vi "Regular Waves (DAQmx).vi"(0 "Run":bool, 1 "Wave Period":dbl(slide)=1.0 min=0.5 max=5.0 step=0.01 scale=0.5..5.0 scale format="%.1f", 2 "Wave Height":dbl(slide)=0.1 min=0.0 step=0.001 scale=0.0..0.2869843515506789 scale format="%.3f") -> ()   [LabVIEW 2012]
uses:
  <vilib>/Analysis/1siggen.llb/Ramp Pattern by Samples.vi
  <vilib>/Analysis/NI_AALBase.lvlib
panel:
  out "Waveform Graph":dbl[](graph)
  out "Waveform Chart":dbl[][](graph)
  in  "Measure Waves":bool
  in  "Settings":bool
  in  "Power":bool
  out "Buffer Size":i32=4000
  # "Regular Wave Generator"
  # "s"
  # "m"
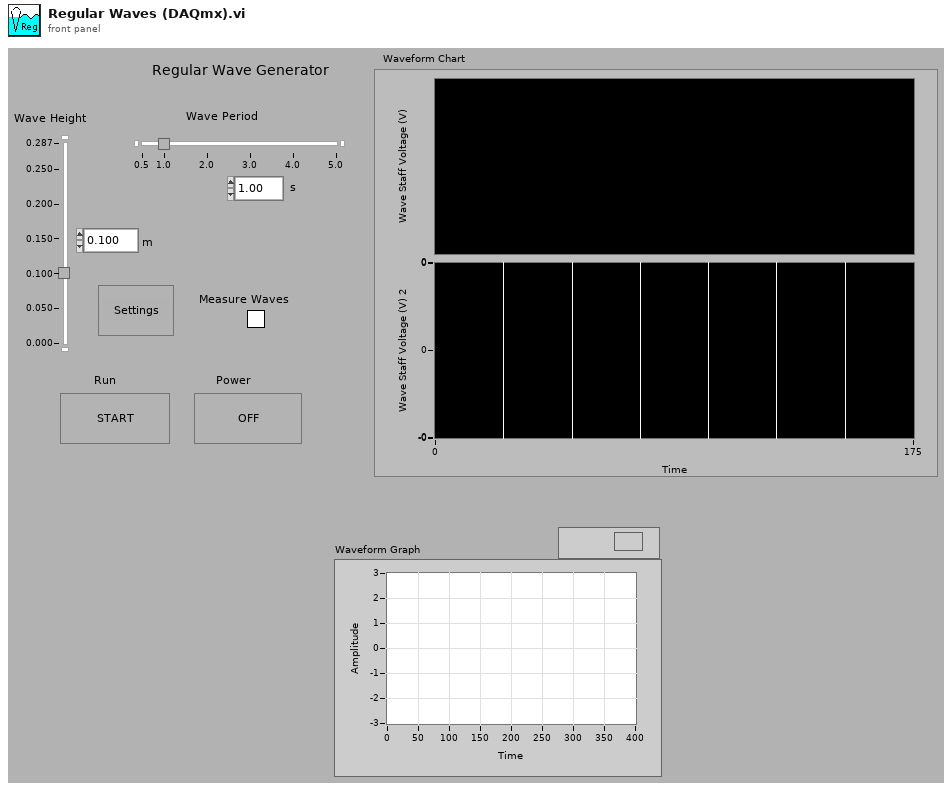
[diagram p1: front panel]
types:
  T1 = cluster{"Output Device":i16, "Output Channel":string, "Sampling Rate (Hz)":dbl, "Input Device":i16, "Input Channel":string, "Input Offset (V)":dbl, "Input Calibration (m/V)":dbl, "Stroke Calibration (V/m)":dbl, "Paddle Height (m)":dbl, "Water Depth (m)":dbl, "Min Period":dbl, "Max Period":dbl, "Max 1/2 Piston Stroke":dbl, "Max H/L":dbl, "Max H/d":dbl}
  T2 = cluster{"Period":dbl, "Wave Height":dbl, "Phase Angle (rad)":dbl}
  T3 = cluster{"Sampling Rate":i32, "Water Depth":dbl, "Paddle Height":dbl}
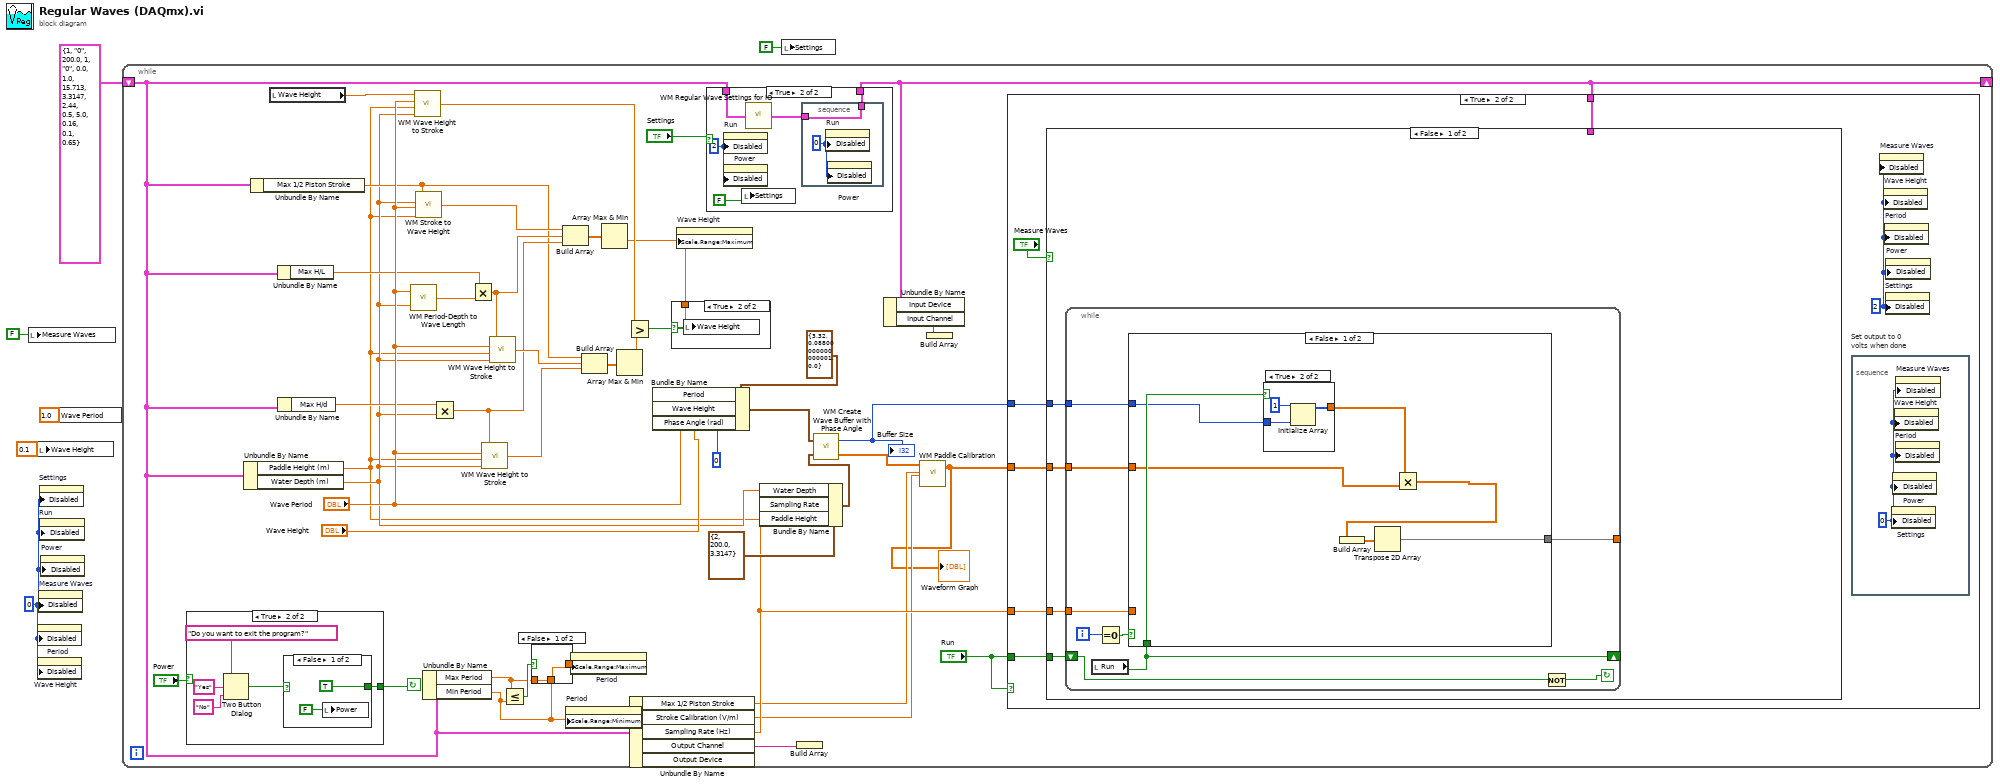
[diagram p0: block diagram]
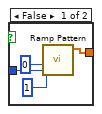
[diagram p3: hidden frame]
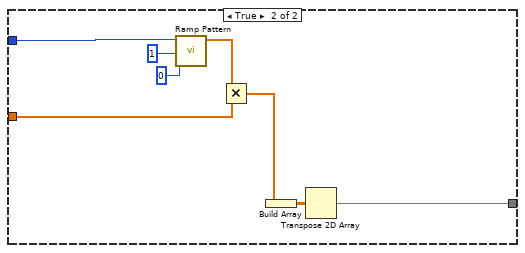
[diagram p4: hidden frame]
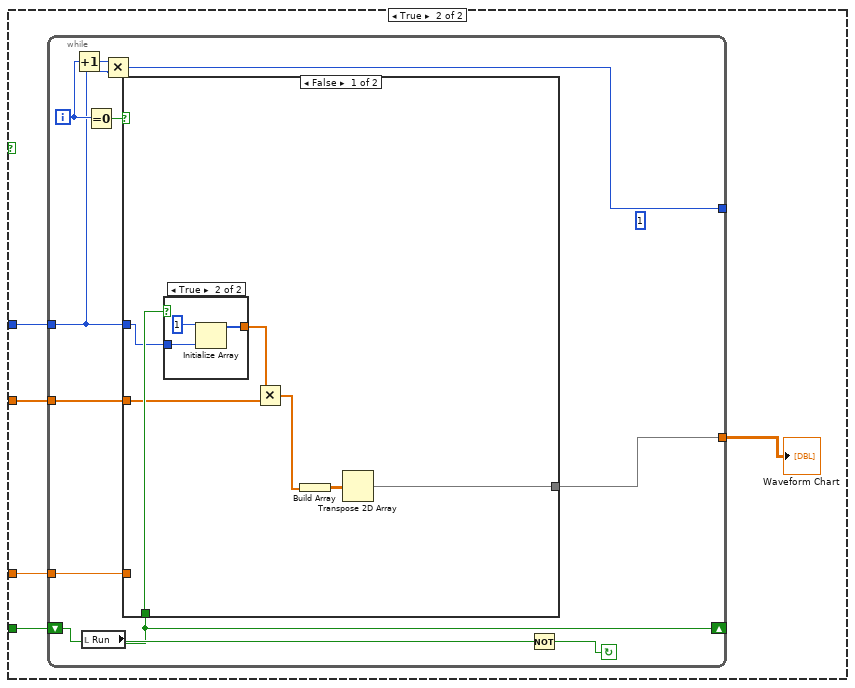
[diagram p5: hidden frame]
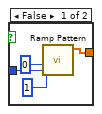
[diagram p6: hidden frame]
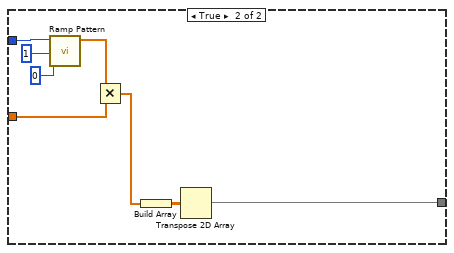
[diagram p7: hidden frame]
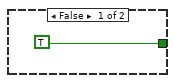
[diagram p9: hidden frame]
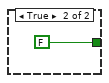
[diagram p10: hidden frame]
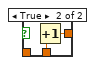
[diagram p11: hidden frame]
diagram:
  w2 = u8 0 ("Write Attribute")
  n1 = local write "Measure Waves"(FALSE ("Measure Waves")) -> ()
  n2 = local write "Wave Height"(0.1 ("Wave Height")) -> ()
  n3 = property on="Period" class="Slide (strict)"("Disabled"=w2) -> ()  [unwired: 2 in, 2 out]
  n4 = property on="Wave Height" class="Slide (strict)"("Disabled"=w2) -> ()  [unwired: 2 in, 2 out]
  n5 = property on="Measure Waves" class="Bool (strict)"("Disabled"=w2) -> ()  [unwired: 2 in, 2 out]
  n6 = property on="Settings" class="Bool (strict)"("Disabled"=w2) -> ()  [unwired: 2 in, 2 out]
  n7 = property on="Run" class="Bool (strict)"("Disabled"=w2) -> ()  [unwired: 2 in, 2 out]
  n8 = property on="Power" class="Bool (strict)"("Disabled"=w2) -> ()  [unwired: 2 in, 2 out]
  n9 = local write "Wave Period"(1.0 ("Period")) -> ()
  n10 = while {
    shift-left: T1 {"Output Device"=1, "Output Channel"="0", "Sampling Rate (Hz)"=200.0, "Input Device"=1, "Input Channel"="0", "Input Offset (V)"=0.0, "Input Calibration (m/V)"=1.0, "Stroke Calibration (V/m)"=15.713, "Paddle Height (m)"=3.3147, "Water Depth (m)"=2.44, "Min Period"=0.5, "Max Period"=5.0, "Max 1/2 Piston Stroke"=0.16, "Max H/L"=0.1, "Max H/d"=0.65} ("Settings") -> [w15]
    shift-right: [w9] -> _
    stop <- w35 continue-if-true
    n11 = case shown="True" "Power" {
      tunnel: [TRUE w140] -> w35
      frame False {
      }
      frame True {
        n12 = Two Button Dialog(message="Do you want to exit the program?", 1:"No" ("F button name (\"Cancel\")"), 2:"Yes" ("T button name (\"OK\")")) -> (T button?=w141:bool)
        n13 = case shown="False" w141 {
          tunnel: [TRUE FALSE] -> w140
          frame False {
            n14 = local write "Power"(FALSE ("Power")) -> ()
          }
          frame True {
          }
        }
      }
    }
    n15 = Unbundle By Name(w15) -> ("Paddle Height (m)"=w18:dbl, "Water Depth (m)"=w19:dbl)
    n16 = Unbundle By Name(w15) -> ("Max 1/2 Piston Stroke"=w22:dbl)
    n17 = local read "Wave Height"() -> (w38:dbl)
    n18 = Unbundle By Name(w15) -> ("Max H/L"=w21:dbl)
    n19 = Unbundle By Name(w15) -> ("Max H/d"=w20:dbl)
    n20 = call "WM Period-Depth to Wave Length.vi"("Water Depth"=w19, "Period"="Wave Period") -> ("WaveLength"=w28:dbl)
    n21 = call "WM Wave Height to Stroke.vi"("Water Depth (m)"=w19, "Flap Height (m)"=w18, "Wave Period (s)"="Wave Period", "Wave Height (m)"=w38) -> ("Flap Amplitude (from x=0) (m)"=w47:dbl)
    n22 = call "WM Stroke to Wave Height.vi"("Paddle Height (m)"=w18, "Wave Period (s)"="Wave Period", "Water Depth (m)"=w19, "Flap Amplitude from x=0 (m)"=w22) -> ("Wave Height (m)"=w42:dbl)
    n23 = Unbundle By Name(w15) -> ("Max Period"=w14:dbl, "Min Period"=w13:dbl)
    n24 = Multiply(x=w20, y=w19) -> (x*y=w27:dbl)
    n25 = Multiply(x=w21, y=w28) -> (x*y=w43:dbl)
    n26 = call "WM Wave Height to Stroke.vi"("Water Depth (m)"=w19, "Flap Height (m)"=w18, "Wave Period (s)"="Wave Period", "Wave Height (m)"=w27) -> ("Flap Amplitude (from x=0) (m)"=w41:dbl)
    n27 = call "WM Wave Height to Stroke.vi"("Water Depth (m)"=w19, "Flap Height (m)"=w18, "Wave Period (s)"="Wave Period", "Wave Height (m)"=w43) -> ("Flap Amplitude (from x=0) (m)"=w40:dbl)
    n28 = Less Or Equal?(x=w14, y=w13) -> (x <= y?=w48:bool)
    n29 = case shown="False" w48 {
      tunnel: w13 -> [_ w150]
      tunnel: [w148 w149] -> w37
      tunnel: w14 -> [w148 _]
      frame False {
      }
      frame True {
        n30 = Increment(x=w150) -> (x+1=w149:dbl)
      }
    }
    n31 = Build Array(w42, w43, w27) -> (w46:dbl[])
    n32 = property on="Period" class="Slide (strict)"("Scale.Range:Minimum"=w13) -> ()  [unwired: 2 in, 2 out]
    n33 = property on="Period" class="Slide (strict)"("Scale.Range:Maximum"=w37) -> ()  [unwired: 2 in, 2 out]
    n34 = Build Array(w22, w40, w41) -> (w45:dbl[])
    n35 = Array Max & Min(array=w46) -> (min value=w39:dbl)  [unwired: 3 out]
    n36 = Array Max & Min(array=w45) -> (min value=w44:dbl)  [unwired: 3 out]
    n37 = Greater?(x=w47, y=w44) -> (0:w49:bool)
    n38 = Unbundle By Name(w15) -> ("Max 1/2 Piston Stroke"=w17:dbl, "Stroke Calibration (V/m)"=w16:dbl, "Sampling Rate (Hz)"=w24:dbl, "Output Channel"=w23:string)  [unwired: 1 out]
    n39 = Bundle By Name(cluster=T2 {"Period"=3.32, "Wave Height"=0.08800000000000001, "Phase Angle (rad)"=0.0} ("Sine Paramaters"), "Period"="Wave Period", "Wave Height"="Wave Height", "Phase Angle (rad)"=0) -> (w31:T2)
    n40 = case shown="True" w49 {
      tunnel: w39 -> [_ w151]
      frame False {
      }
      frame True {
        n41 = local write "Wave Height"(w151) -> ()
      }
    }
    n42 = property on="Wave Height" class="Slide (strict)"("Scale.Range:Maximum"=w39) -> ()  [unwired: 2 in, 2 out]
    n43 = case shown="True" "Settings" {
      tunnel: w15 -> [w131 w136]
      tunnel: [w131 w134] -> w9
      frame False {
      }
      frame True {
        w132 = u8 2 ("Write Attribute")
        n44 = property on="Run" class="Bool (strict)"("Disabled"=w132) -> ()  [unwired: 2 in, 2 out]
        n45 = property on="Power" class="Bool (strict)"("Disabled"=w132) -> ()  [unwired: 2 in, 2 out]
        n46 = local write "Settings"(FALSE ("Settings")) -> ()
        n47 = call "WM Regular Wave Settings for IO.vi"("Settings"=w136) -> ("Settings Output"=w135:T1)
        n48 = stacked-sequence {
          tunnel: w135 -> [w138]
          tunnel: [w138] -> w134
          frame #0 {
            w137 = u8 0 ("Write Attribute")
            n49 = property on="Run" class="Bool (strict)"("Disabled"=w137) -> ()  [unwired: 2 in, 2 out]
            n50 = property on="Power" class="Bool (strict)"("Disabled"=w137) -> ()  [unwired: 2 in, 2 out]
          }
        }
      }
    }
    n51 = Bundle By Name(cluster=T3 {"Sampling Rate"=2, "Water Depth"=200.0, "Paddle Height"=3.3147} ("Buffer Info"), "Water Depth"=w19, "Sampling Rate"=w24, "Paddle Height"=w18) -> (w33:T3)
    n52 = Build Array(w23) -> ()  [unwired: 1 out]
    n53 = call "WM Create Wave Buffer with Phase Angle.vi"("Buffer Info"=w33, "Sine Paramaters"=w31) -> ("Output"=w8:dbl[], "Buffer Size"=w11:i32)
    "Buffer Size" <- w11
    n54 = Unbundle By Name(w9) -> ("Input Channel"=w12:string)  [unwired: 1 out]
    n55 = call "WM Paddle Calibration.vi"("Stroke Calibration (V/m)"=w16, "Max 1/2 Piston Stroke (m)"=w17, "Input Stroke Distance (m)"=w8) -> ("Output Voltage"=w7:dbl[])  [unwired: 1 in, 1 out]
    "Waveform Graph" <- w7
    n56 = Build Array(w12) -> ()  [unwired: 1 out]
    n57 = case shown="True" "Run" {
      tunnel: w11 -> [_ w56]
      tunnel: "Run" -> [_ w55]
      tunnel: w7 -> [_ w54]
      tunnel: w24 -> [_ w53]
      tunnel: w9 -> [_ w50]
      frame False {
      }
      frame True {
        w51 = u8 2 ("Write Attribute")
        n58 = case shown="False" "Measure Waves" {
          tunnel: w56 -> [w60 w96]
          tunnel: w55 -> [w59 w94]
          tunnel: w54 -> [w58 w95]
          tunnel: w53 -> [w57 w93]
          tunnel: w50 -> [_ _]
          frame False {
            n59 = while {
              tunnel: w60 -> [w64]
              tunnel: w58 -> [w65]
              tunnel: w57 -> [w66]
              shift-left: w59 -> [w67]
              shift-right: [w63] -> _
              tunnel: [w61] -> _
              i -> [w69]
              stop <- w62 continue-if-true
              n60 = local read "Run"() -> (w63:bool)
              n61 = Equal To 0?(x=w69) -> (x = 0?=w68:bool)
              n62 = case shown="False" w68 {
                tunnel: w66 -> [_ _]
                tunnel: w63 -> [w75 _]
                tunnel: w65 -> [w73 w86]
                tunnel: w64 -> [w72 w87]
                tunnel: [w70 w84] -> w61
                frame False {
                  n63 = case shown="True" w75 {
                    tunnel: [w80 w81] -> w76
                    tunnel: w72 -> [w77 w83]
                    frame False {
                      n64 = call-poly <vilib>:"Ramp Pattern.vi"("start"=1, "end"=0, "samples"=w77) -> ("Ramp Pattern"=w80:dbl[])  [unwired: 7 in, 1 out]
                    }
                    frame True {
                      n65 = Initialize Array(1, w83) -> (w81:i32[])
                    }
                  }
                  n66 = Multiply(x=w76, y=w73) -> (x*y=w71:dbl[])
                  n67 = Build Array(w71) -> (w74:dbl[][])
                  n68 = Transpose 2D Array(2D array=w74) -> (transposed array=w70:dbl[][])
                }
                frame True {
                  n69 = call-poly <vilib>:"Ramp Pattern.vi"("start"=0, "end"=1, "samples"=w87) -> ("Ramp Pattern"=w88:dbl[])  [unwired: 7 in, 1 out]
                  n70 = Multiply(x=w88, y=w86) -> (x*y=w85:dbl[])
                  n71 = Build Array(w85) -> (w91:dbl[][])
                  n72 = Transpose 2D Array(2D array=w91) -> (transposed array=w84:dbl[][])
                }
              }
              n73 = Not(x=w67) -> (.not. x?=w62:bool)
            }
          }
          frame True {
            (unwired) 1 ("Dimension Size")
            n74 = while {
              tunnel: [w99] -> _
              tunnel: w96 -> [w100]
              tunnel: w95 -> [w104]
              tunnel: w93 -> [w105]
              shift-left: w94 -> [w106]
              shift-right: [w103] -> _
              tunnel: [w97] -> w92
              i -> [w102]
              stop <- w98 continue-if-true
              n75 = Increment(x=w102) -> (x+1=w101:i32)
              n76 = local read "Run"() -> (w103:bool)
              n77 = Equal To 0?(x=w102) -> (x = 0?=w107:bool)
              n78 = Multiply(x=w101, y=w100) -> (x*y=w99:i32)
              n79 = case shown="False" w107 {
                tunnel: w105 -> [_ _]
                tunnel: w103 -> [w113 _]
                tunnel: w104 -> [w111 w125]
                tunnel: w100 -> [w109 w123]
                tunnel: [w108 w122] -> w97
                frame False {
                  n80 = case shown="True" w113 {
                    tunnel: [w118 w119] -> w114
                    tunnel: w109 -> [w115 w121]
                    frame False {
                      n81 = call-poly <vilib>:"Ramp Pattern.vi"("start"=1, "end"=0, "samples"=w115) -> ("Ramp Pattern"=w118:dbl[])  [unwired: 7 in, 1 out]
                    }
                    frame True {
                      n82 = Initialize Array(1, w121) -> (w119:i32[])
                    }
                  }
                  n83 = Multiply(x=w114, y=w111) -> (x*y=w110:dbl[])
                  n84 = Build Array(w110) -> (w112:dbl[][])
                  n85 = Transpose 2D Array(2D array=w112) -> (transposed array=w108:dbl[][])
                }
                frame True {
                  n86 = call-poly <vilib>:"Ramp Pattern.vi"("start"=0, "end"=1, "samples"=w123) -> ("Ramp Pattern"=w126:dbl[])  [unwired: 7 in, 1 out]
                  n87 = Multiply(x=w126, y=w125) -> (x*y=w124:dbl[])
                  n88 = Build Array(w124) -> (w129:dbl[][])
                  n89 = Transpose 2D Array(2D array=w129) -> (transposed array=w122:dbl[][])
                }
              }
              n90 = Not(x=w106) -> (.not. x?=w98:bool)
            }
            "Waveform Chart" <- w92
          }
        }
        n91 = stacked-sequence "Set output to 0\nvolts when done" {
          frame #0 {
            w130 = u8 0 ("Write Attribute")
            n92 = property on="Settings" class="Bool (strict)"("Disabled"=w130) -> ()  [unwired: 2 in, 2 out]
            n93 = property on="Power" class="Bool (strict)"("Disabled"=w130) -> ()  [unwired: 2 in, 2 out]
            n94 = property on="Wave Height" class="Slide (strict)"("Disabled"=w130) -> ()  [unwired: 2 in, 2 out]
            n95 = property on="Period" class="Slide (strict)"("Disabled"=w130) -> ()  [unwired: 2 in, 2 out]
            n96 = property on="Measure Waves" class="Bool (strict)"("Disabled"=w130) -> ()  [unwired: 2 in, 2 out]
          }
        }
        n97 = property on="Measure Waves" class="Bool (strict)"("Disabled"=w51) -> ()  [unwired: 2 in, 2 out]
        n98 = property on="Wave Height" class="Slide (strict)"("Disabled"=w51) -> ()  [unwired: 2 in, 2 out]
        n99 = property on="Period" class="Slide (strict)"("Disabled"=w51) -> ()  [unwired: 2 in, 2 out]
        n100 = property on="Settings" class="Bool (strict)"("Disabled"=w51) -> ()  [unwired: 2 in, 2 out]
        n101 = property on="Power" class="Bool (strict)"("Disabled"=w51) -> ()  [unwired: 2 in, 2 out]
      }
    }
  }
  n102 = local write "Settings"(FALSE ("Settings")) -> ()
